vi "Read Default Value.vi"(8 "error in (no error)":errorcluster, 11 "Boolean Data Type in":refnum<class "Boolean Data Type.lvclass">) -> (0 "error out":errorcluster, 2 "Default Value":string, 3 "Boolean Data Type out":refnum<class "Boolean Data Type.lvclass">)   [LabVIEW 2018, in "Boolean Data Type.lvclass"]
uses:
  Boolean Data Type.lvclass
  Boolean Data Type.lvclass/Boolean Data Type.ctl
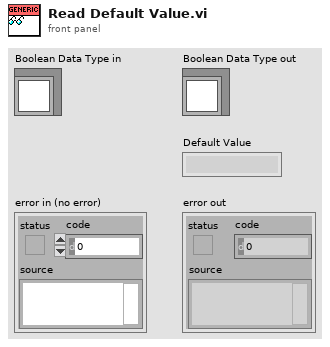
[diagram p1: front panel]
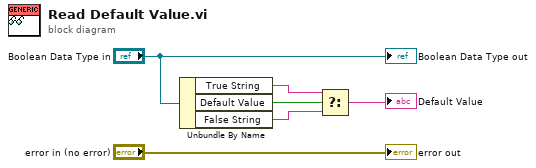
[diagram p0: block diagram]
diagram:
  n1 = Unbundle By Name("Boolean Data Type in") -> ("True String"=w3:string, "Default Value"=w4:bool, "False String"=w2:string)
  n2 = Select(t=w3, s=w4, f=w2) -> (s? t:f=→"Default Value":string)
  "error out" <- "error in (no error)"
  "Boolean Data Type out" <- "Boolean Data Type in"
